vi "AutoHoldCan.vi"(10 "Store Trashcan?":bool) -> ()   [LabVIEW 2014]
uses:
  Robot Global Data.vi
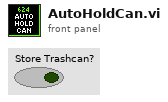
[diagram p1: front panel]
types:
  T1 = typedef "Elevator Control Command.ctl" = cluster{"Command":T2, "Manual Motor Out":dbl, "Manual Eject Piston":bool, "Mode":T3, "Override Limits":bool, "Manual Stabilizer":bool, "Manual Finger":bool, "Store Trashcan?":bool, "Hold Low?":bool, "Idle Mode":T4, "HP Load":bool, "Unstick":bool}
  T2 = typedef "Elevator Command.ctl" = enum16{"Idle", "Load 1", "Load 2", "Load 3", "Drop Stack", "Eject Stack", "Untip Trashcan", "Load Trashcan", "HP Load", "HP Score"}
  T3 = typedef "Elevator Mode.ctl" = enum16{"Manual", "Safe", "Auto"}
  T4 = typedef "Elevator Idle Mode.ctl" = enum16{"Load 1", "Load 2", "Load 3", "Load Can", "Untip Can", "Step Load", "Drop Stack"}
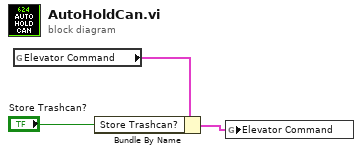
[diagram p0: block diagram]
diagram:
  n1 = global read "Robot Global Data.vi" "Elevator Command"() -> (w3:T1)
  n2 = Bundle By Name(cluster=w3, "Store Trashcan?"="Store Trashcan?") -> (w1:T1)
  n3 = global write "Robot Global Data.vi" "Elevator Command"(w1) -> ()
